vi "LedMain.vi"(8 "error in (no error)":errorcluster, 10 "Mode":enum16{"Open", "Run"}(ring)) -> (0 "error out (no error)":errorcluster)   [LabVIEW 2016]
uses:
  <vilib>/Rock Robotics/WPI/SerialPort/WPI_SerialPort.ctl
panel:
  in  "Serial Port":T1
  # "2017 LED Main Control VI\nFRC Team 34"
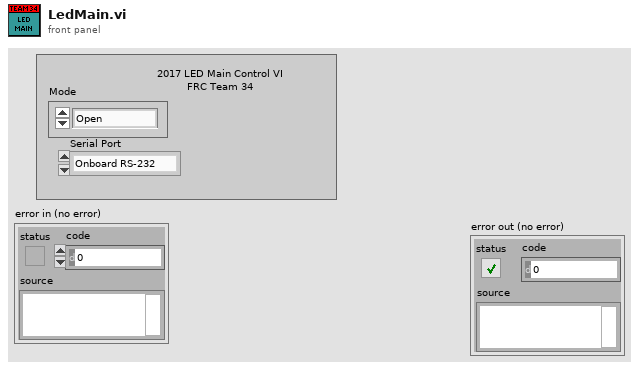
[diagram p1: front panel]
types:
  T1 = typedef "WPI_SerialPort.ctl" = enum16{"Onboard RS-232", "MXP TTL", "USB 1", "USB 2"}
  T2 = enum16{"Alliance", "Demo", "Police", "Train", "Climb"}
  T3 = typedef "WPI_SerialPortRef.ctl" = cluster{"DevStatus":errorcluster, "Serial Port Name":refnum<visa-resource-name>}
  T4 = typedef "WPI_SwitchDevRef.ctl" = cluster{"DevStatus":errorcluster, "DIO Channel":T5, "CntIndex":T6, "Normally Closed":bool}
  T5 = typedef "FPGA_DIOChannel.ctl" = enum8{"DIO 0", "DIO 1", "DIO 2", "DIO 3", "DIO 4", "DIO 5", "DIO 6", "DIO 7", "DIO 8", "DIO 9", "DIO MXP 0", "DIO MXP 1", "DIO MXP 2", "DIO MXP 3", "DIO MXP 4", "DIO MXP 5", "DIO MXP 6", "DIO MXP 7", "DIO MXP 8", "DIO MXP 9", "DIO MXP 10", "DIO MXP 11", "DIO MXP 12", "DIO MXP 13", "DIO MXP 14", "DIO MXP 15", "SPI Port CS1", "SPI Port CS2", "SPI Port CS3", "SPI Port MISO", "SPI Port MOSI", "Invalid"}
  T6 = typedef "FPGA_CounterCtrSystemIndex.ctl" = enum8{"Ctr 0", "Ctr 1", "Ctr 2", "Ctr 3", "Ctr 4", "Ctr 5", "Ctr 6", "Ctr 7", "Invalid"}
  T7 = typedef "WPI_DriverStationAllianceInfo.ctl" = enum16{"Red", "Blue", "Invalid"}
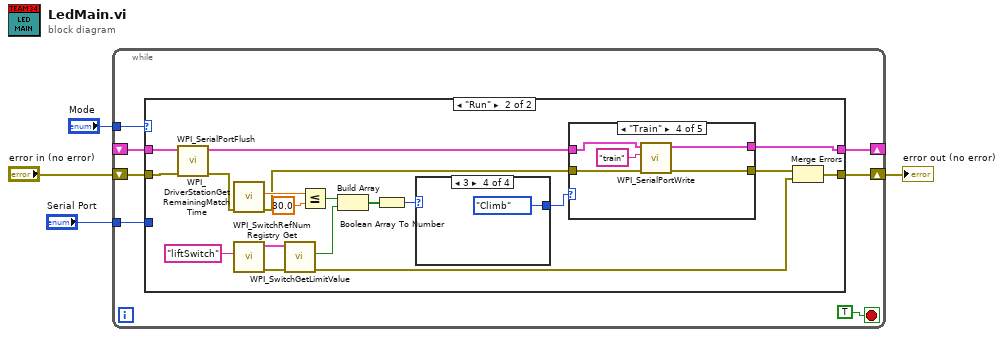
[diagram p0: block diagram]
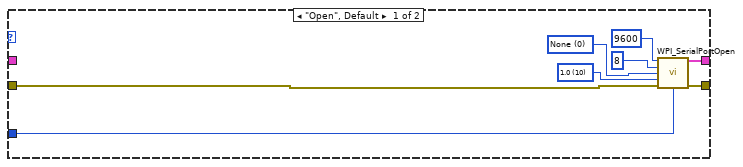
[diagram p2: hidden frame]
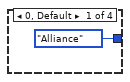
[diagram p3: hidden frame]
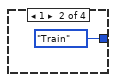
[diagram p4: hidden frame]
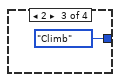
[diagram p5: hidden frame]
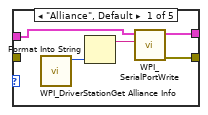
[diagram p6: hidden frame]
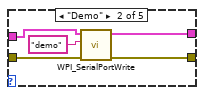
[diagram p7: hidden frame]
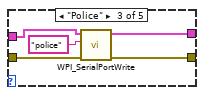
[diagram p8: hidden frame]
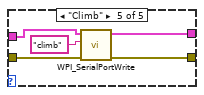
[diagram p9: hidden frame]
diagram:
  n1 = while {
    tunnel: "Mode" -> [w11]
    shift-right: [w9] -> w2
    shift-left: "error in (no error)" -> [w8]
    shift-right: [w7] -> _
    shift-left: _ -> [w5]
    tunnel: "Serial Port" -> [w6]
    stop <- TRUE stop-if-true
    n2 = case shown="\"Run\"" w11 {
      tunnel: w8 -> [w15 w37]
      tunnel: [w14 w22] -> w9
      tunnel: [w13 w35] -> w7
      tunnel: w6 -> [w12 _]
      tunnel: w5 -> [_ w38]
      frame "Open", Default {
        w16 = u16 10 items=["1.0"=10, "1.5"=15, "2.0"=20] ("Stop Bits")
        w17 = u16 0 items=["None", "Odd", "Even", "Mark", "Space"] ("Parity")
        n3 = call <vilib>:"WPI_SerialPortOpen.vi"("Baud Rate"=u32 9600, "Data Bits"=u16 8, "Parity"=w17, "Stop Bits"=w16, "error in (no error)"=w15, "Serial Port"=w12) -> ("SerialPortRef"=w13:T3, "error out"=w14:errorcluster)  [unwired: 8 in]
      }
      frame "Run" {
        n4 = call <vilib>:"WPI_SerialPortFlush.vi"("error in (no error)"=w37, "SerialPortRef"=w38) -> ("error out"=w33:errorcluster, "SerialPortRef"=w36:T3)  [unwired: 8 in]
        n5 = call <vilib>:"WPI_DriverStationGetRemainingMatchTime.vi"("error in (no error)"=w33) -> ("error out"=w32:errorcluster, "Match Time(s)"=w34:sgl)  [unwired: 9 in]
        n6 = call <vilib>:"WPI_SwitchRefNum Registry Get.vi"("refnum name"="liftSwitch") -> ("error out"=w24:errorcluster, "SwitchDevRef"=w25:T4)  [unwired: 9 in]
        n7 = call <vilib>:"WPI_SwitchGetLimitValue.vi"("error in (no error)"=w24, "SwitchDevRef"=w25) -> ("error out"=w20:errorcluster, "Switch Pressed"=w21:bool)  [unwired: 7 in, 1 out]
        n8 = Less Or Equal?(x=w34, y=sgl 30.0) -> (x <= y?=w30:bool)
        n9 = Build Array(w30, w21) -> (w29:bool[])
        n10 = Boolean Array To Number(Boolean array=w29) -> (number=w28:u32)
        n11 = case shown="3" w28 {
          tunnel: [T2."Alliance" T2."Train" T2."Climb" T2."Climb"] -> w27
          frame 0, Default {
          }
          frame 1 {
          }
          frame 2 {
          }
          frame 3 {
          }
        }
        n12 = case shown="\"Train\"" w27 {
          tunnel: w36 -> [w47 w52 w54 w59 w67]
          tunnel: [w46 w50 w57 w61 w65] -> w23
          tunnel: [w45 w51 w56 w60 w66] -> w35
          tunnel: w32 -> [_ w49 w55 w62 w64]
          frame "Alliance", Default {
            n13 = call <vilib>:"WPI_DriverStationGet Alliance Info.vi"() -> ("Alliance"=w44:T7)  [unwired: 10 in, 1 out]
            n14 = Format Into String(w44) -> (resulting string=w43:string)  [unwired: 3 in, 1 out]
            n15 = call <vilib>:"WPI_SerialPortWrite.vi"("Buffer"=w43, "SerialPortRef"=w47) -> ("error out"=w46:errorcluster, "SerialPortRef"=w45:T3)  [unwired: 7 in, 1 out]
          }
          frame "Demo" {
            n16 = call <vilib>:"WPI_SerialPortWrite.vi"("error in (no error)"=w49, "Buffer"="demo", "SerialPortRef"=w52) -> ("error out"=w50:errorcluster, "SerialPortRef"=w51:T3)  [unwired: 6 in, 1 out]
          }
          frame "Police" {
            n17 = call <vilib>:"WPI_SerialPortWrite.vi"("error in (no error)"=w55, "Buffer"="police", "SerialPortRef"=w54) -> ("error out"=w57:errorcluster, "SerialPortRef"=w56:T3)  [unwired: 6 in, 1 out]
          }
          frame "Train" {
            n18 = call <vilib>:"WPI_SerialPortWrite.vi"("error in (no error)"=w62, "Buffer"="train", "SerialPortRef"=w59) -> ("error out"=w61:errorcluster, "SerialPortRef"=w60:T3)  [unwired: 6 in, 1 out]
          }
          frame "Climb" {
            n19 = call <vilib>:"WPI_SerialPortWrite.vi"("error in (no error)"=w64, "Buffer"="climb", "SerialPortRef"=w67) -> ("error out"=w65:errorcluster, "SerialPortRef"=w66:T3)  [unwired: 6 in, 1 out]
          }
        }
        n20 = Merge Errors(w23, w20) -> (w22:errorcluster)
      }
    }
  }
  "error out (no error)" <- w2
